vi "zero accellerometer routine.vi"(7 "add reading":bool, 10 "accel":cluster{"x":dbl, "y":dbl, "z":dbl}, 11 "accel range":T1) -> (1 "y offset":dbl, 2 "x offset":dbl, 3 "accel range out":T1)   [LabVIEW 2017]
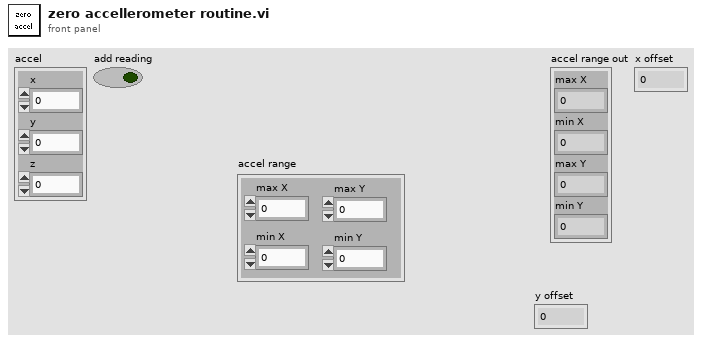
[diagram p1: front panel]
types:
  T1 = cluster{"max X":dbl, "min X":dbl, "max Y":dbl, "min Y":dbl}
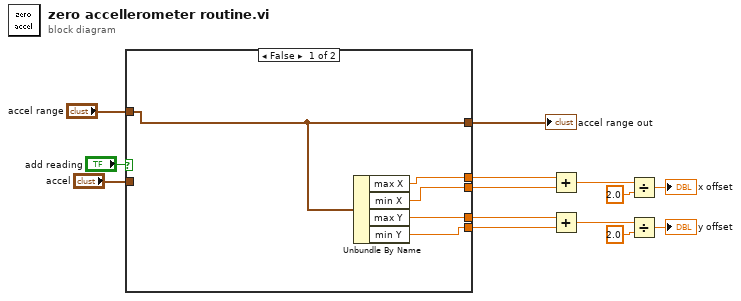
[diagram p0: block diagram]
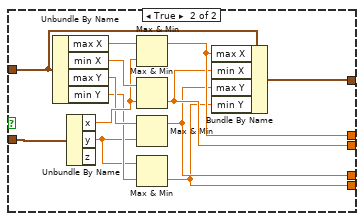
[diagram p2: hidden frame]
diagram:
  n1 = case shown="False" "add reading" {
    tunnel: "accel" -> [_ w32]
    tunnel: [w19 w26] -> w13
    tunnel: "accel range" -> [w19 w25]
    tunnel: [w18 w24] -> w11
    tunnel: [w17 w23] -> w10
    tunnel: [w16 w22] -> w3
    tunnel: [w15 w21] -> w2
    frame False {
      n2 = Unbundle By Name(w19) -> ("max X"=w18:dbl, "min X"=w17:dbl, "max Y"=w16:dbl, "min Y"=w15:dbl)
    }
    frame True {
      n3 = Unbundle By Name(w25) -> ("max X"=w31:dbl, "min X"=w30:dbl, "max Y"=w28:dbl, "min Y"=w27:dbl)
      n4 = Unbundle By Name(w32) -> ("x"=w29:dbl, "y"=w20:dbl)  [unwired: 1 out]
      n5 = Max & Min(x=w31, y=w29) -> (max(x,y)=w24:dbl)  [unwired: 1 out]
      n6 = Max & Min(x=w30, y=w29) -> (min(x,y)=w23:dbl)  [unwired: 1 out]
      n7 = Max & Min(x=w28, y=w20) -> (max(x,y)=w22:dbl)  [unwired: 1 out]
      n8 = Max & Min(x=w20, y=w27) -> (min(x,y)=w21:dbl)  [unwired: 1 out]
      n9 = Bundle By Name(cluster=w25, "max X"=w24, "min X"=w23, "max Y"=w22, "min Y"=w21) -> (w26:T1)
    }
  }
  "accel range out" <- w13
  n10 = Add(x=w11, y=w10) -> (x+y=w9:dbl)
  n11 = Add(x=w3, y=w2) -> (x+y=w6:dbl)
  n12 = Divide(x=w9, y=2.0) -> (x/y=→"x offset":dbl)
  n13 = Divide(x=w6, y=2.0) -> (x/y=→"y offset":dbl)
